vi "Auto_corr.vi"(8 "m":i32=3, 9 "P":i32=9, 11 "input A":dbl[](array[numeric])=[1.0, 3.0, 5.0, 6.0, 1.0, 9.0, 0.0, 7.0, 4.0, 3.0, 9.0, 6.0, 1.0, 0.0, 0.0, 3.0, 8.0, 9.0, 2.0, 4.0, 5.0, 5.0, 1.0, 2.0, 0.0, 2.0, 3.0, 2.0, 1.0, 1.0, 0.0, 9.0, 8.0, 7.0, 4.0, 1.0, 1.0, 8.0, 9.0]) -> (0 "Sn":dbl[](array[numeric]), 3 "Acc":dbl[](array[numeric]))   [LabVIEW 2015]
panel:
  out "size(s)":i32
  out "ceil(x): smallest int >= x":dbl
  out "shift register":dbl[](array[numeric])
  out "Numeric":i32
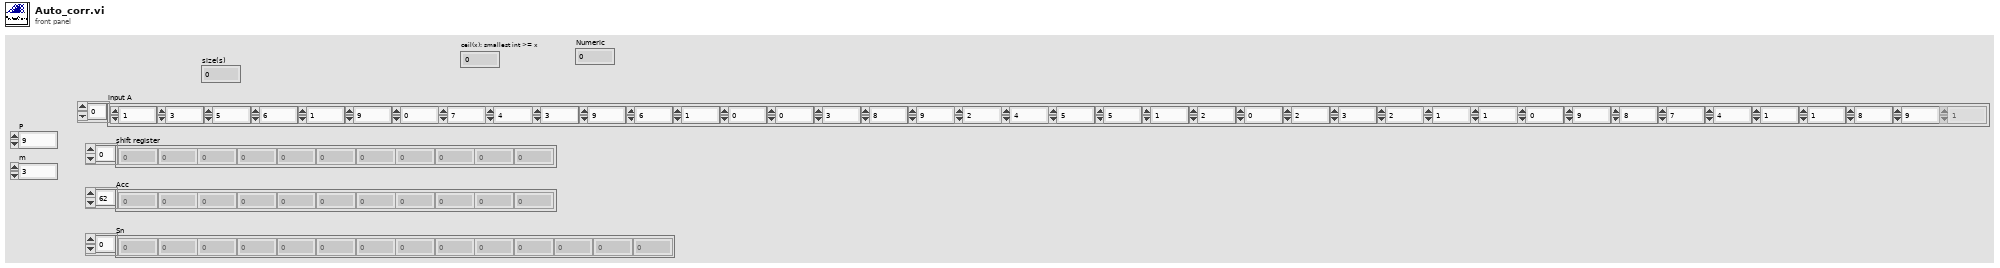
[diagram p1: front panel]
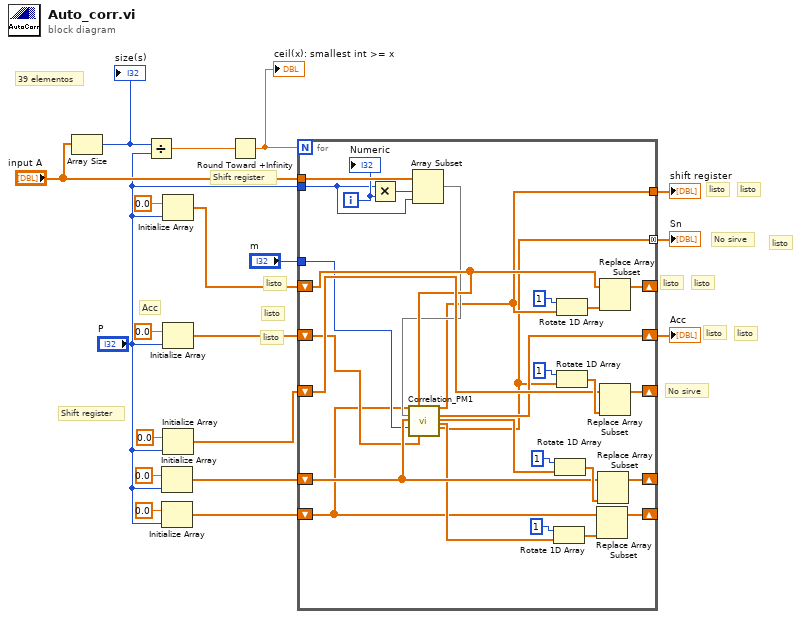
[diagram p0: block diagram]
diagram:
  # "No sirve"
  # "listo"
  # "listo"
  # "listo"
  # "listo"
  # "listo"
  # "listo"
  # "listo"
  # "No sirve"
  # "listo"
  # "listo"
  # "listo"
  # "Shift register"
  # "Acc"
  # "Shift register"
  # "39 elementos"
  n1 = Array Size(array="input A") -> (size(s)=w18:i32)
  "size(s)" <- w18
  n2 = Divide(x=w18, y="P") -> (x/y=w17:dbl)
  n3 = Initialize Array(0.0 ("dimension size"), "P") -> (w4:dbl[])
  n4 = Initialize Array(0.0 ("dimension size"), "P") -> (w2:dbl[])
  n5 = Initialize Array(0.0 ("dimension size"), "P") -> (w7:dbl[])
  n6 = Initialize Array(0.0 ("dimension size"), "P") -> (w6:dbl[])
  n7 = Initialize Array(0.0 ("dimension size"), "P") -> (w5:dbl[])
  n8 = Round Toward +Infinity(x=w17) -> (ceil(x): smallest int >= x=w16:dbl)
  "ceil(x): smallest int >= x" <- w16
  n9 = for {
    N: w16 -> [_]
    tunnel: "P" -> [w34]
    tunnel: "m" -> [w30]
    shift-right: [w45] -> _
    shift-left: w7 -> [w33]
    shift-right: [w22] -> w11
    shift-left: w6 -> [w29]
    tunnel: [w23] -> w15
    tunnel: "input A" -> [w44]
    tunnel: [w20] -> w10 mode=concatenating
    shift-right: [w40] -> _
    shift-left: w5 -> [w39]
    shift-right: [w36] -> _
    shift-left: w4 -> [w31]
    shift-right: [w26] -> _
    shift-left: w2 -> [w24]
    i -> [w35]
    n10 = Multiply(x=w34, y=w35) -> (x*y=w43:i32)
    n11 = Array Subset(array=w44, index=w43, length=w34) -> (w32:dbl[])
    n12 = call "Correlation_PM1.vi"("shift register D"=w24, "Input A"=w32, "shift register MY"=w31, "m"=w30, "shift register in"=w33, "Acc in"=w29) -> ("shift register"=w23:dbl[], "Acc"=w22:dbl[], "shift register Y out"=w21:dbl[], "shift register D out"=w25:dbl[], "MnA"=w20:dbl[])  [unwired: 17 in]
    n13 = Rotate 1D Array(1:w25, 2:1 ("n")) -> (0:w27:dbl[])
    n14 = Rotate 1D Array(1:w21, 2:1 ("n")) -> (0:w37:dbl[])
    n15 = Rotate 1D Array(1:w23, 2:1 ("n")) -> (0:w46:dbl[])
    n16 = Rotate 1D Array(1:w20, 2:1 ("n")) -> (0:w41:dbl[])
    n17 = Replace Array Subset(array=w24, new element=w27) -> (w26:dbl[])  [unwired: 1 in]
    n18 = Replace Array Subset(array=w31, new element=w37) -> (w36:dbl[])  [unwired: 1 in]
    n19 = Replace Array Subset(array=w33, new element=w46) -> (w45:dbl[])  [unwired: 1 in]
    n20 = Replace Array Subset(array=w39, new element=w41) -> (w40:dbl[])  [unwired: 1 in]
    "Numeric" <- w35
  }
  "shift register" <- w15
  "Acc" <- w11
  "Sn" <- w10
